vi "Get Shift Values.vi"(8 "error in (no error)":errorcluster, 11 "AVI Path":path) -> (0 "error out":errorcluster)   [LabVIEW 2012]
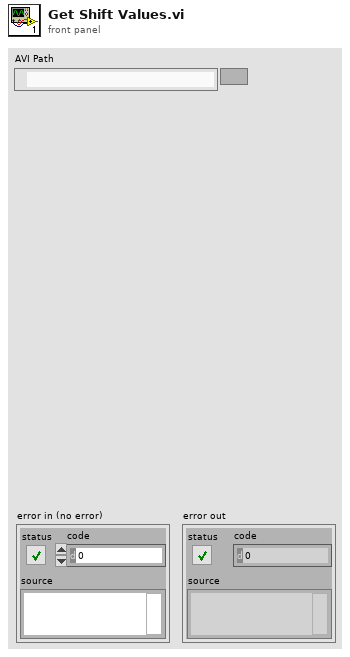
[diagram p1: front panel]
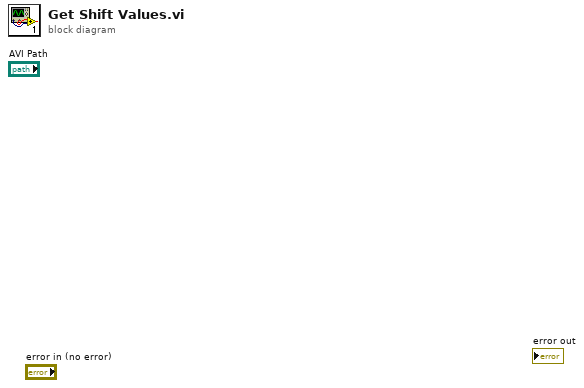
[diagram p0: block diagram]
diagram:
